vi "Status__LCR.vi"(7 "Action (Get)":enum16{"Get", "Set", "Reset"}(ring), 10 "Status In":u16 format="%.0b", 11 "Bit":u16) -> (2 "Status Out":u16 format="%.0b", 3 "Bit Value Out":bool)   [LabVIEW 2011, in "BooleanXControl__LCR.xctl"]
doc: "This VI will perform bit-wise actions.\n<b>Reset</b>: Resets the specified bit to false\n<b>Set</b>: Sets the specified bit to true\n<b>Get</b>: Reads the boolean value of the specified bit (Default action)"
uses:
  BooleanXControl__LCR.xctl
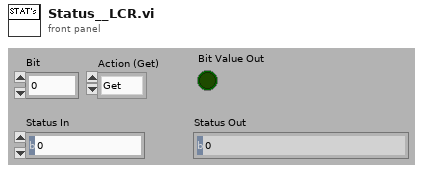
[diagram p1: front panel]
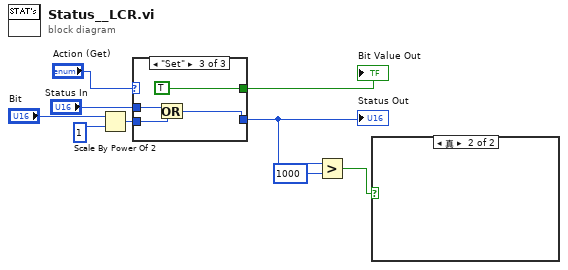
[diagram p0: block diagram]
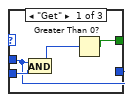
[diagram p3: hidden frame]
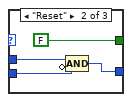
[diagram p4: hidden frame]
diagram:
  n1 = Scale By Power Of 2(n="Bit", x=u16 1) -> (x*2^n=w7:u16)
  n2 = case shown="\"Set\"" "Action (Get)" {
    tunnel: "Status In" -> [w10 w16 w21]
    tunnel: w7 -> [w13 w15 w20]
    tunnel: [w10 w14 w19] -> w3
    tunnel: [w11 FALSE TRUE] -> w6
    frame "Get" {
      n3 = And(x=w10, y=w13) -> (x .and. y?=w12:u16)
      n4 = Greater Than 0?(x=w12) -> (x > 0?=w11:bool)
    }
    frame "Reset" {
      n5 = Compound Arithmetic op=AND(w16, invert w15) -> (w14:u16)
    }
    frame "Set" {
      n6 = Or(x=w21, y=w20) -> (x .or. y?=w19:u16)
    }
  }
  "Status Out" <- w3
  "Bit Value Out" <- w6
  n7 = Greater?(x=w3, y=u16 1000) -> (0:w1:bool)
  n8 = case shown="真" w1 {
    frame False {
    }
    frame True {
    }
  }
